vi "waveformsAObuffer.vi"(1 "AO wf in":waveform(dbl)[](array[waveform]), 2 "command":string="clear") -> (0 "AO wf out":waveform(dbl)[](array[waveform]))   [LabVIEW 2015]
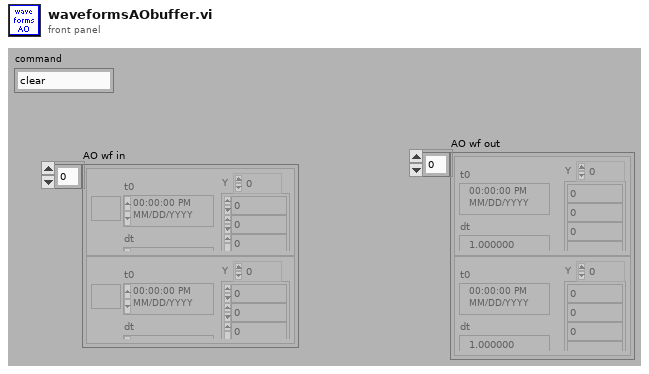
[diagram p1: front panel]
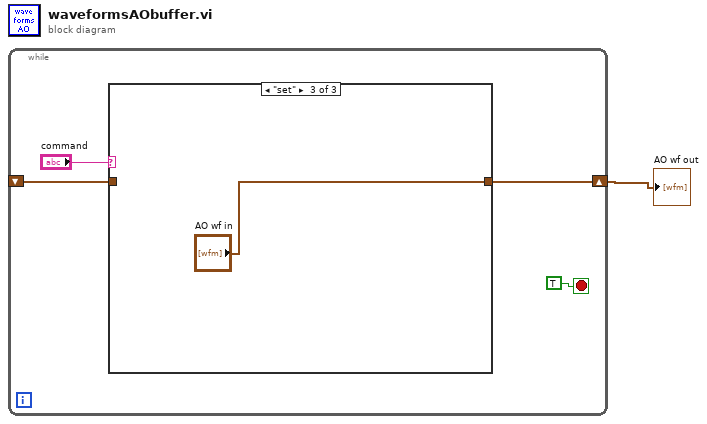
[diagram p0: block diagram]
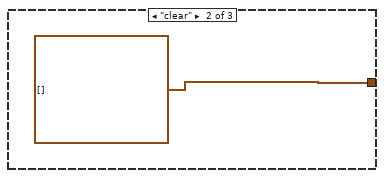
[diagram p3: hidden frame]
diagram:
  n1 = while {
    shift-right: [w3] -> w1
    shift-left: _ -> [w2]
    stop <- TRUE stop-if-true
    n2 = case shown="\"set\"" "command" {
      tunnel: [w6 waveform(dbl)[] [] ("Analog waveforms") "AO wf in"] -> w3
      tunnel: w2 -> [w6 _ _]
      frame "get", Default {
      }
      frame "clear" {
      }
      frame "set" {
      }
    }
  }
  "AO wf out" <- w1
